vi "AlliGator Sliced Mean, SDV & CV Enter Data Dialog.vi"(8 "Error In":errorcluster, 10 "X min":dbl, 11 "X max":dbl) -> (0 "Error Out":errorcluster, 1 "Cancelled?":bool, 3 "Slices Definition out":T1={"Axis Start"=0.0, "Axis Stop"=0.0, "# Steps"=0, "Step Size"=1.0, "Step Definition"=enum."# Steps", "Upper Percentile"=1.0, "Lower Percentile"=1.0, "Min # Data Points/Slice"=1, "Output Abscissa Statistics Plots"=FALSE, "Bin Location"=enum."Left", "# Elements"=1, "Bootstrap CV's SDV"=FALSE, "# Replicas"=1} {"# Replicas" min=1; "# Elements" min=0; "Min # Data Points/Slice" min=0 max=100; "Lower Percentile" min=0.0 max=100.0; "Upper Percentile" min=0.0 max=100.0; "Step Size" min=1.0; "# Steps" min=1})   [LabVIEW 2021, in "AlliGator Lifetime & Other Parameters.lvlib"]
uses:
  AlliGator Lifetime & Other Parameters.lvlib
  Graphs/XY Graph/XY Graph Sliced Mean & SDV Step Definition.ctl
  AlliGator Intensity Slice Definition.ctl
  Graphs/XY Graph/XY Graph Sliced CV Abscissa Location.ctl
  Graphs/XY Graph/XY Graph Add-Ons.lvlib
panel:
  in  "Use Data Min/Max":bool
  in  "Slices Definition":T1={"Axis Start"=0.0, "Axis Stop"=0.0, "# Steps"=1, "Step Size"=1.0, "Step Definition"=enum."# Steps", "Upper Percentile"=100.0, "Lower Percentile"=0.0, "Min # Data Points/Slice"=1, "Output Abscissa Statistics Plots"=FALSE, "Bin Location"=enum."Mean", "# Elements"=1, "Bootstrap CV's SDV"=FALSE, "# Replicas"=1} {"# Replicas" min=1; "# Elements" min=1; "Min # Data Points/Slice" min=1; "Lower Percentile" min=0.0 max=100.0; "Upper Percentile" min=0.0 max=100.0; "Step Size" min=0.0; "# Steps" min=1}
  out "Message":string="Enter the first (start) and last (stop) values to consider for the analysis, as well as the number of intervals (# Steps) in which to divide the range of values:"
  in  "Cancel":bool
  in  "OK":bool
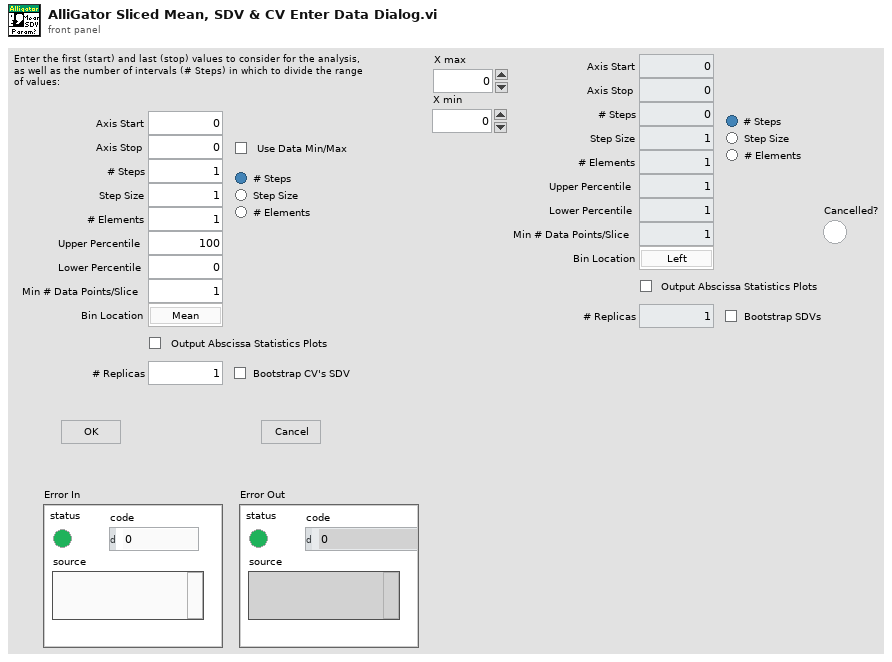
[diagram p1: front panel]
types:
  T1 = typedef "XY Graph Add-Ons.lvlib/XY Graph Sliced Mean & SDV Step Definition.ctl" = cluster{"Axis Start":dbl, "Axis Stop":dbl, "# Steps":i32, "Step Size":dbl, "Step Definition":T2, "Upper Percentile":dbl, "Lower Percentile":dbl, "Min # Data Points/Slice":i32, "Output Abscissa Statistics Plots":bool, "Bin Location":T3, "# Elements":i32, "Bootstrap CV's SDV":bool, "# Replicas":i32}
  T2 = typedef "AlliGator Lifetime & Other Parameters.lvlib/AlliGator Intensity Slice Definition.ctl" = enum32{"# Steps", "Step Size", "# Elements"}
  T3 = typedef "XY Graph Add-Ons.lvlib/XY Graph Sliced CV Abscissa Location.ctl" = enum16{"Left", "Center", "Mean", "Right"}
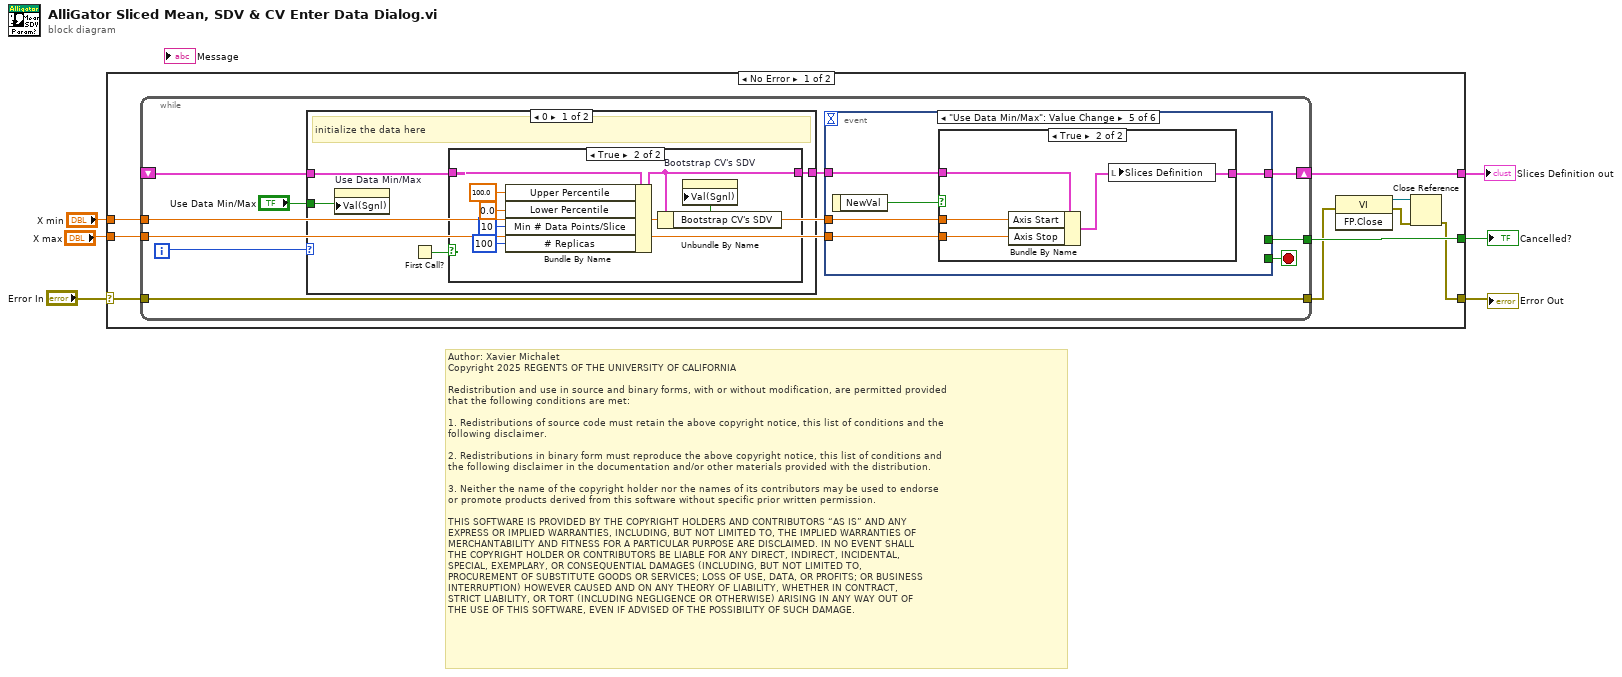
[diagram p0: block diagram]
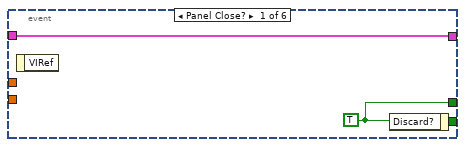
[diagram p4: hidden frame]
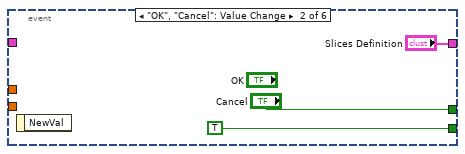
[diagram p5: hidden frame]
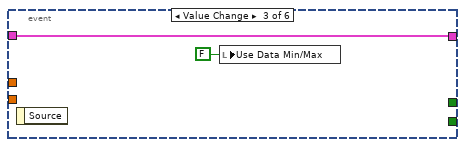
[diagram p6: hidden frame]
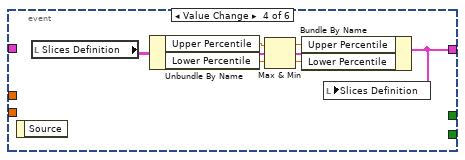
[diagram p7: hidden frame]
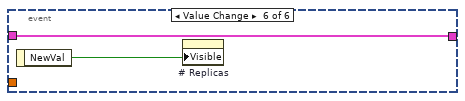
[diagram p9: hidden frame]
diagram:
  # "Author: Xavier Michalet\nCopyright 2025 REGENTS OF THE UNIVERSITY OF CALIFORNIA\n\nRedistribution and use in source and binary forms, with or without modification, are permitted provided\nthat the following conditions are met:\n\n1. Redistributions of source code must retain the above copyright notice, this list of conditions and the\nfollowing disclaimer.\n\n2. Redistributions in binary form must reproduce the above copyright notice, this list of conditions and\nthe following disclaimer in the documentation and/or other materials provided with the distribution.\n\n3. Neither the name of the copyright holder nor the names of its contributors may be used to endorse \nor promote products derived from this software without specific prior written permission.\n\nTHIS SOFTWARE IS PROVIDED BY THE COPYRIGHT HOLDERS AND CONTRIBUTORS “AS IS” AND ANY \nEXPRESS OR IMPLIED WARRANTIES, INCLUDING, BUT NOT LIMITED TO, THE IMPLIED WARRANTIES OF\nMERCHANTABILITY AND FITNESS FOR A PARTICULAR PURPOSE ARE DISCLAIMED. IN NO EVENT SHALL\nTHE COPYRIGHT HOLDER OR CONTRIBUTORS BE LIABLE FOR ANY DIRECT, INDIRECT, INCIDENTAL, \nSPECIAL, EXEMPLARY, OR CONSEQUENTIAL DAMAGES (INCLUDING, BUT NOT LIMITED TO, \nPROCUREMENT OF SUBSTITUTE GOODS OR SERVICES; LOSS OF USE, DATA, OR PROFITS; OR BUSINESS\nINTERRUPTION) HOWEVER CAUSED AND ON ANY THEORY OF LIABILITY, WHETHER IN CONTRACT, \nSTRICT LIABILITY, OR TORT (INCLUDING NEGLIGENCE OR OTHERWISE) ARISING IN ANY WAY OUT OF\nTHE USE OF THIS SOFTWARE, EVEN IF ADVISED OF THE POSSIBILITY OF SUCH DAMAGE."
  n1 = case shown="No Error" "Error In" {
    selector: "Error In" -> [w10 w64]
    tunnel: [w15 _] -> w6
    tunnel: [w14 _] -> w3
    tunnel: [w11 w64] -> w4
    tunnel: "X min" -> [w8 _]
    tunnel: "X max" -> [w7 _]
    frame No Error {
      n2 = while {
        tunnel: [w24] -> w15
        shift-right: [w21] -> w14
        shift-left: _ -> [w22]
        tunnel: w10 -> [w19]
        tunnel: [w19] -> w9
        tunnel: w8 -> [w18]
        tunnel: w7 -> [w17]
        i -> [w23]
        stop <- w25 stop-if-true
        n3 = case shown="0" w23 {
          tunnel: w22 -> [w27 w38]
          tunnel: [w28 w38] -> w20
          tunnel: "Use Data Min/Max" -> [w26 _]
          frame 0 {
            # "initialize the data here"
            n4 = property on="Use Data Min/Max" class="Bool (strict)"("Val(Sgnl)"=w26) -> ()  [unwired: 2 in, 2 out]
            n5 = First Call?() -> (First Call?: T/F=w29:bool)
            n6 = case shown="True" w29 {
              tunnel: w27 -> [w30 w37]
              tunnel: [w30 w32] -> w28
              frame False {
              }
              frame True {
                n7 = Bundle By Name(cluster=w37, "Upper Percentile"=100.0, "Lower Percentile"=0.0, "Min # Data Points/Slice"=10, "# Replicas"=100) -> (w32:T1)
                n8 = Unbundle By Name(w32) -> ("Bootstrap CV's SDV"=w31:bool)
                n9 = property on="Bootstrap CV's SDV" class="Bool (strict)"("Val(Sgnl)"=w31) -> ()  [unwired: 2 in, 2 out]
              }
            }
          }
          frame 1, Default {
          }
        }
        n10 = event shown="[4] \"Use Data Min/Max\": Value Change" {
          selector: _ -> [_ _ _ _ _ _]
          dyn-events: _ -> [_ _ _ _ _ _]
          timeout: _ -> [_ _ _ _ _ _]
          tunnel: [w40 TRUE ("Discard?") _ _ _ _] -> w25
          tunnel: [w40 "Cancel" _ _ _ _] -> w24
          tunnel: [w39 "Slices Definition" w44 w46 w53 w62] -> w21
          tunnel: w20 -> [w39 _ w44 _ w56 w62]
          tunnel: w18 -> [_ _ _ _ w55 _]
          tunnel: w17 -> [_ _ _ _ w54 _]
          event Panel Close? {
            w40 = TRUE ("Discard?")
            n11 = event-data() -> ()  [unwired: 1 in, 1 out]
            n12 = event-data("Discard?"=w40) -> ()  [unwired: 1 in, 1 out]
          }
          event "OK", "Cancel": Value Change {
            n13 = event-data() -> ()  [unwired: 1 in, 1 out]
          }
          event Value Change {
            n14 = event-data() -> ()  [unwired: 1 in, 1 out]
            n15 = local write "Use Data Min/Max"(FALSE ("Use Data Min/Max")) -> ()
          }
          event Value Change {
            n16 = event-data() -> ()  [unwired: 1 in, 1 out]
            n17 = local read "Slices Definition"() -> (w49:T1)
            n18 = Unbundle By Name(w49) -> ("Upper Percentile"=w51:dbl, "Lower Percentile"=w50:dbl)
            n19 = Max & Min(x=w51, y=w50) -> (max(x,y)=w48:dbl, min(x,y)=w47:dbl)
            n20 = Bundle By Name(cluster=w49, "Upper Percentile"=w48, "Lower Percentile"=w47) -> (w46:T1)
            n21 = local write "Slices Definition"(w46) -> ()
          }
          event "Use Data Min/Max": Value Change {
            n22 = event-data() -> ("NewVal"=w52:bool)  [unwired: 1 in]
            n23 = case shown="True" w52 {
              tunnel: w56 -> [w57 w61]
              tunnel: w55 -> [_ w60]
              tunnel: w54 -> [_ w59]
              tunnel: [w57 w58] -> w53
              frame False {
              }
              frame True {
                n24 = Bundle By Name(cluster=w61, "Axis Start"=w60, "Axis Stop"=w59) -> (w58:T1)
                n25 = local write "Slices Definition"(w58) -> ()
              }
            }
          }
          event Value Change {
            n26 = event-data() -> ("NewVal"=w63:bool)  [unwired: 1 in]
            n27 = property on="# Replicas" class="DigNum (strict)"("Visible"=w63) -> ()  [unwired: 2 in, 2 out]
          }
        }
      }
      n28 = invoke class="VI" method="FP.Close"(error in=w9) -> (reference out=w13:refnum<vi>, error out=w12:errorcluster)  [unwired: 2 in, 1 out]
      n29 = Close Reference(reference=w13, error in (no error)=w12) -> (error out=w11:errorcluster)
    }
    frame Error {
    }
  }
  "Cancelled?" <- w6
  "Error Out" <- w4
  "Slices Definition out" <- w3
